vi "EMV T6 Offset From Target.vi"(8 "error in (no error)":errorcluster, 9 "T6_OFFSET_FROM_TARGET_INDICATING_FLOW":dbl=3.0, 10 "User Setpoint Temperature":u16=125, 11 "Mixing Valve.T6 Temp (0x406E) in":dbl) -> (0 "error out":errorcluster, 3 "Flow Dectection":bool)   [LabVIEW 2016]
panel:
  out "Absolute T6 Offset From Target":dbl
  out "T6 History":dbl[](array[numeric])
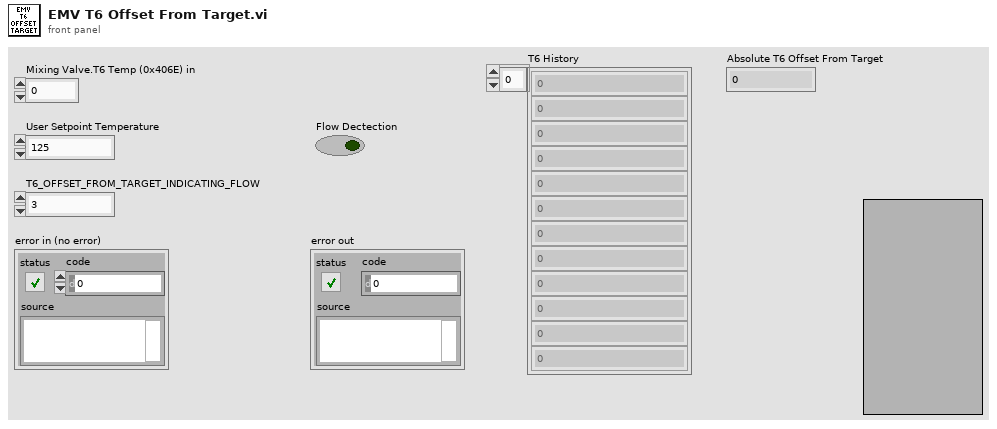
[diagram p1: front panel]
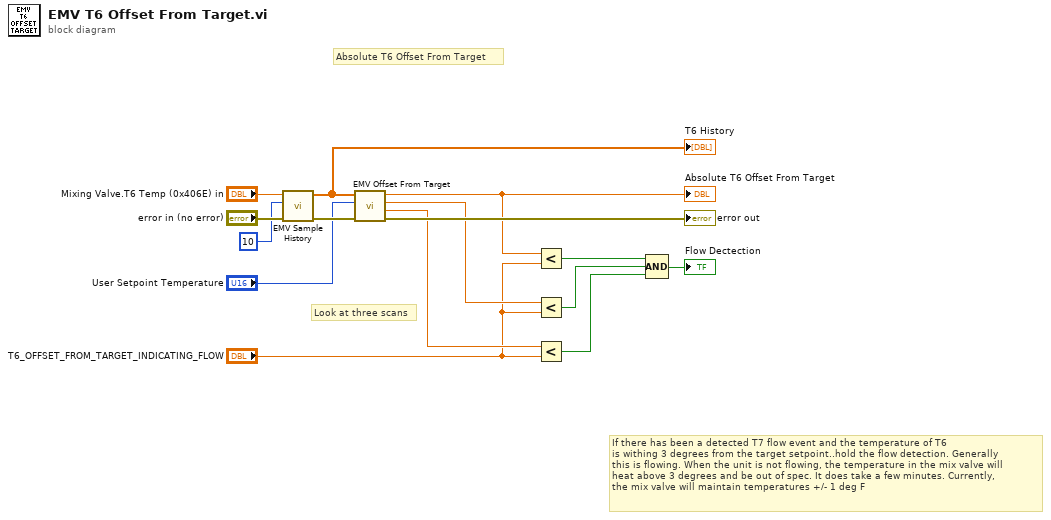
[diagram p0: block diagram]
diagram:
  # "Look at three scans"
  # "If there has been a detected T7 flow event and the temperature of T6 \nis withing 3 degrees from the target setpoint..hold the flow detection. Generally\nthis is flowing. When the unit is not flowing, the temperature in the mix valve will \nheat above 3 degrees and be out of spec. It does take a few minutes. Currently,\nthe mix valve will maintain temperatures +/- 1 deg F"
  # "Absolute T6 Offset From Target"
  n1 = call "EMV Sample History.vi"("error in (no error)"="error in (no error)", "length"=10, "T6 Temp"="Mixing Valve.T6 Temp (0x406E) in") -> ("error out"=w13:errorcluster, "T6 History"=w14:dbl[])  [unwired: 7 in]
  "T6 History" <- w14
  n2 = call "EMV Offset From Target.vi"("error in (no error)"=w13, "User Setpoint Temperature"="User Setpoint Temperature", "Current T6 Temperatures"=w14) -> ("error out"=→"error out":errorcluster, "Absolute T6 Offset From Target 3"=w7:dbl, "Absolute T6 Offset From Target 2"=w8:dbl, "Absolute T6 Offset From Target 1"=w10:dbl)  [unwired: 5 in]
  "Absolute T6 Offset From Target" <- w10
  n3 = Less?(x=w10, y="T6_OFFSET_FROM_TARGET_INDICATING_FLOW") -> (x < y?=w5:bool)
  n4 = Less?(x=w8, y="T6_OFFSET_FROM_TARGET_INDICATING_FLOW") -> (x < y?=w4:bool)
  n5 = Less?(x=w7, y="T6_OFFSET_FROM_TARGET_INDICATING_FLOW") -> (x < y?=w3:bool)
  n6 = Compound Arithmetic op=AND(w5, w4, w3) -> (→"Flow Dectection":bool)
